vi "Fetch Sensor Identifiers .vi"(7 "Message":string="Fetch Model Numbers", 8 "error in (no error)":errorcluster, 10 "SQL Statement":string="SELECT ModelNumber FROM TestConfigurations", 11 "Database in":refnum<queue>) -> (0 "error out":errorcluster, 2 "Sensors Results":string[](array[string]), 3 "Database out":refnum<queue>)   [LabVIEW 2026, in "Settings.lvlib"]
uses:
  Architecture/Message Queue/Message Cluster.ctl
  controls/Messaging Payloads/DB Query Request Payload.ctl
  Architecture/Message Queue/Enqueue Message (Single).vi
  Settings/Settings.lvlib
  Architecture/Message Queue/Message Queue.lvlib
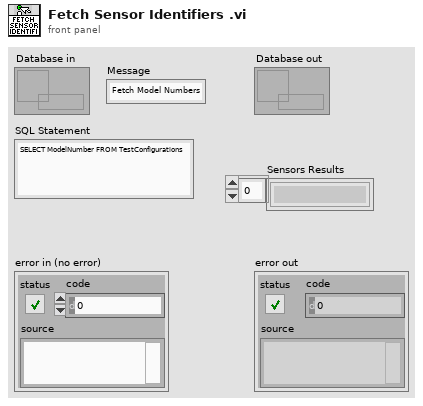
[diagram p1: front panel]
types:
  T1 = typedef "DB Query Request Payload.ctl" = cluster{"SQL Statement":string, "Notifier":refnum<notifier>}
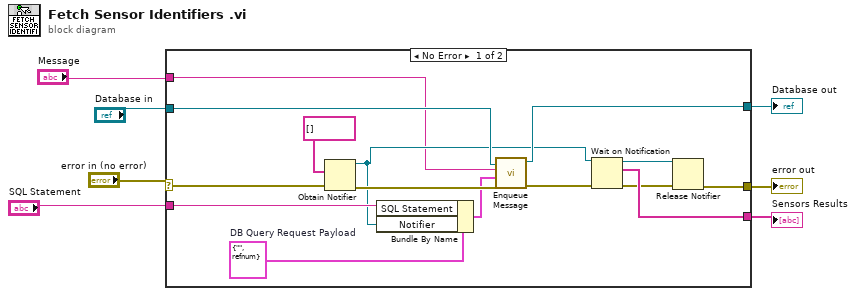
[diagram p0: block diagram]
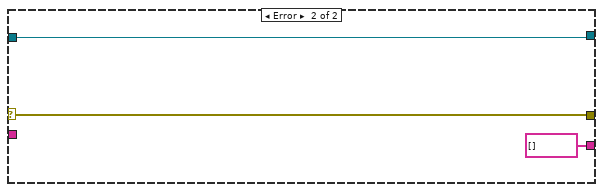
[diagram p2: hidden frame]
diagram:
  n1 = case shown="No Error" "error in (no error)" {
    selector: "error in (no error)" -> [w13 w24]
    tunnel: [w22 string[] []] -> w7
    tunnel: [w21 w25] -> w6
    tunnel: "Database in" -> [w20 w25]
    tunnel: [w19 w24] -> w4
    tunnel: "SQL Statement" -> [w11 _]
    tunnel: "Message" -> [w8 _]
    frame No Error {
      w12 = T1 {"SQL Statement"="", "Notifier"=refnum}  # DB Query Request Payload
      n2 = Obtain Notifier(notification data type=string[] [], error in (no error)=w13) -> (notifier out=w10:refnum<notifier>, error out=w15:errorcluster)  [unwired: 2 in, 1 out]
      n3 = Bundle By Name(cluster=w12, "SQL Statement"=w11, "Notifier"=w10) -> (w9:T1)
      n4 = call-poly "Enqueue Message.vi"("error in (no error)"=w15, "Message Data"=w9, "Message"=w8, "Message Queue"=w20) -> ("error out"=w16:errorcluster, "dup Message Queue"=w21:refnum<queue>)  [unwired: 6 in]
      n5 = Wait on Notification(notifier=w10, error in (no error)=w16) -> (notifier out=w18:refnum<notifier>, notification=w22:string[], error out=w17:errorcluster)  [unwired: 2 in, 1 out]
      n6 = Release Notifier(notifier=w18, error in (no error)=w17) -> (error out=w19:errorcluster)  [unwired: 1 in, 2 out]
    }
    frame Error {
    }
  }
  "Sensors Results" <- w7
  "Database out" <- w6
  "error out" <- w4
